vi "Create New Azure Queue.vi"() -> ()   [LabVIEW 2015]
doc: "Demonstrates how to create a new Azure queue."
uses:
  Core/Azure Credentials.ctl
  Core/Session/Session.lvclass
  Core/NI_Azure_Core.lvlib
  Queue/NI_Azure_Queue.lvlib
panel:
  in  "Access Key":string
  in  "Storage Account Name":string
  in  "Queue Name":string
  # "Overview: Demonstrates how to create a new Azure queue.\nRequirements: NI Cloud Toolkit for Azure and a registered Microsoft Azure account\nInstructions:\n1. Specify the Storage Account Name and Access Key for your Azure account. You can create an account at http://azure.microsoft.com.\n2. Specify a Queue Name for the queue you want to create. Note that queue names can only contain numbers and lowercase letters.\n3. Run the VI. Verify in the Microsoft Azure Portal that the specified queue was created."
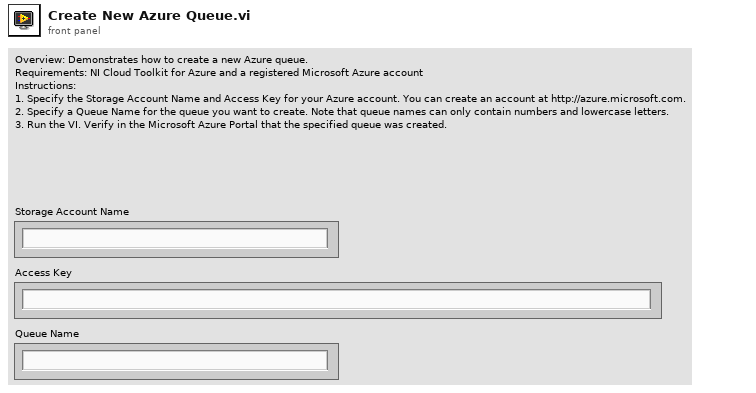
[diagram p1: front panel]
types:
  T1 = typedef "NI_Azure_Core.lvlib/Azure Credentials.ctl" = cluster{"Storage Account Name":string, "Access Key":string}
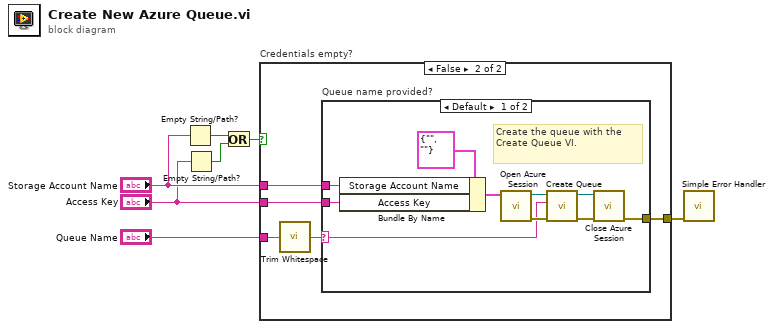
[diagram p0: block diagram]
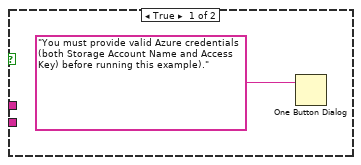
[diagram p2: hidden frame]
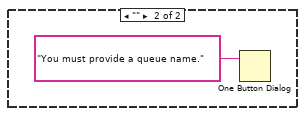
[diagram p3: hidden frame]
diagram:
  n1 = Empty String/Path?(string/path="Storage Account Name") -> (empty?=w7:bool)
  n2 = Empty String/Path?(string/path="Access Key") -> (empty?=w6:bool)
  n3 = Or(x=w7, y=w6) -> (x .or. y?=w5:bool)
  n4 = case "Credentials empty?" shown="False" w5 {
    tunnel: "Storage Account Name" -> [_ w13]
    tunnel: "Access Key" -> [_ w12]
    tunnel: "Queue Name" -> [_ w11]
    tunnel: [_ w9] -> w1
    frame True {
      n5 = One Button Dialog(message="You must provide valid Azure credentials (both Storage Account Name and Access Key) before running this example).") -> ()  [unwired: 1 in, 1 out]
    }
    frame False {
      n6 = call <vilib>:"Trim Whitespace.vi"("string"=w11) -> ("trimmed string"=w10:string)  [unwired: 1 in]
      n7 = case "Queue name provided?" shown="Default" w10 {
        selector: w10 -> [w14 _]
        tunnel: w13 -> [w23 _]
        tunnel: w12 -> [w22 _]
        tunnel: [w15 _] -> w9
        frame Default {
          # "Create the queue with the Create Queue VI."
          n8 = Bundle By Name(cluster=T1 {"Storage Account Name"="", "Access Key"=""} ("Credentials"), "Storage Account Name"=w23, "Access Key"=w22) -> (w21:T1)
          n9 = call "Open Azure Session.vi"("Credentials"=w21) -> ("error out"=w19:errorcluster, "Azure Session"=w18:refnum<class "Session.lvclass">)  [unwired: 9 in]
          n10 = call "Create Queue.vi"("error in (no error)"=w19, "Queue"=w14, "Azure Session in"=w18) -> ("error out"=w16:errorcluster, "Azure Session out"=w17:refnum<class "Session.lvclass">)  [unwired: 7 in]
          n11 = call "Close Azure Session.vi"("error in (no error)"=w16, "Azure Session"=w17) -> ("error out"=w15:errorcluster)  [unwired: 9 in]
        }
        frame "" {
          n12 = One Button Dialog(message="You must provide a queue name.") -> ()  [unwired: 1 in, 1 out]
        }
      }
    }
  }
  n13 = call <vilib>:"Simple Error Handler.vi"("error in (no error)"=w1) -> ()  [unwired: 4 in, 5 out]
